vi "form status alarm string.vi"(0 "Vmon":dbl[][](array[numeric]), 1 "Vset":dbl[][](array[numeric]), 2 "Imon":dbl[][](array[numeric]), 3 "Iset":dbl[][](array[numeric]), 4 "Timestamps":dbl[][](array[numeric]), 5 "error in":errorcluster, 10 "Num Channels Read":i32, 12 "Start index":i32) -> (14 "Error Status String":string, 15 "All channels in error":string, 16 "Error Logged":bool[](array[boolean]), 17 "Error Array":string[][](array[string]), 18 "Status Strings":string[](array[string]), 19 "Error Out":errorcluster)   [LabVIEW 2018]
uses:
  CAEN globals.vi
  <userlib>/_OpenG.lib/array/array.llb/Search 1D Array (Boolean)__ogtk.vi
  <userlib>/_OpenG.lib/array/array.llb/Index 1D Array Elements (Boolean)__ogtk.vi
  <userlib>/_OpenG.lib/array/array.llb/Index 1D Array Elements (DBL)__ogtk.vi
  <userlib>/_OpenG.lib/array/array.llb/Index 1D Array Elements (String)__ogtk.vi
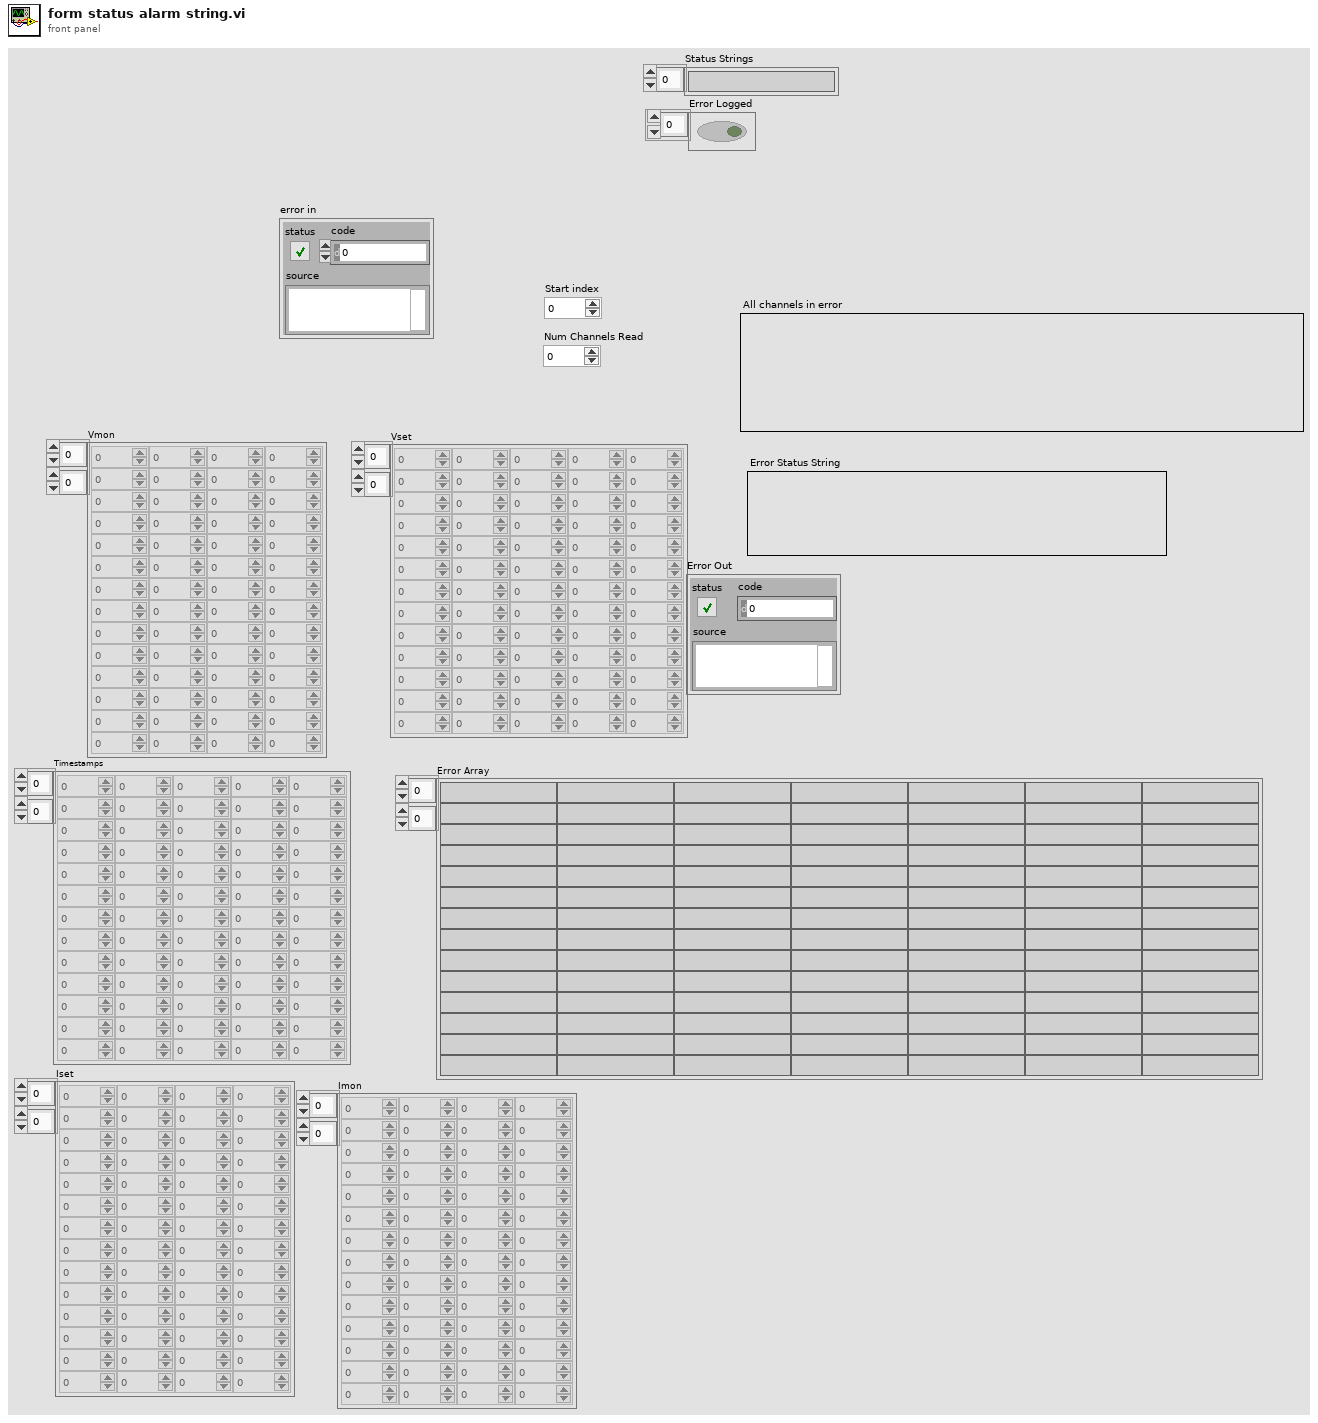
[diagram p1: front panel]
types:
  T1 = cluster{"Crate num":i32, "Slot nums":i32[], "Channel nums":i32[][], "N chans":i32[]}[]
  T2 = typedef "channel_cluster.ctl" = cluster{"Channel Name":string, "Crate":i32, "Card Type":string, "Card":i32, "Channel":i32, "Status Icon":picture, "Vmon (V)":dbl, "Vset (V)":dbl, "Imon (A)":dbl, "Iset (A)":dbl, "Timestamp":string, "ON/OFF":bool, "Status":string, "Vswmax (V)":dbl, "Flag":bool, "Vfile (V)":dbl, "Error Logged":bool[], "enable_file":bool}
  T3 = cluster{"Numeric":i32, "Indices of Elements":i32[], "Indices of Elements":i32[][], "Indices of Elements":i32[]}
  T4 = cluster{"Numeric":i32, "Indices of Elements":i32[], "Indices of Elements":i32[][], "Indices of Elements":i32[]}[]
  T5 = cluster{"Numeric":i32, "Indices of Elements":i32[], i32[][], i32[]}
  T6 = cluster{"Numeric":i32, "Indices of Elements":i32[], "Channel nums":i32[][], "N chans":i32[]}[]
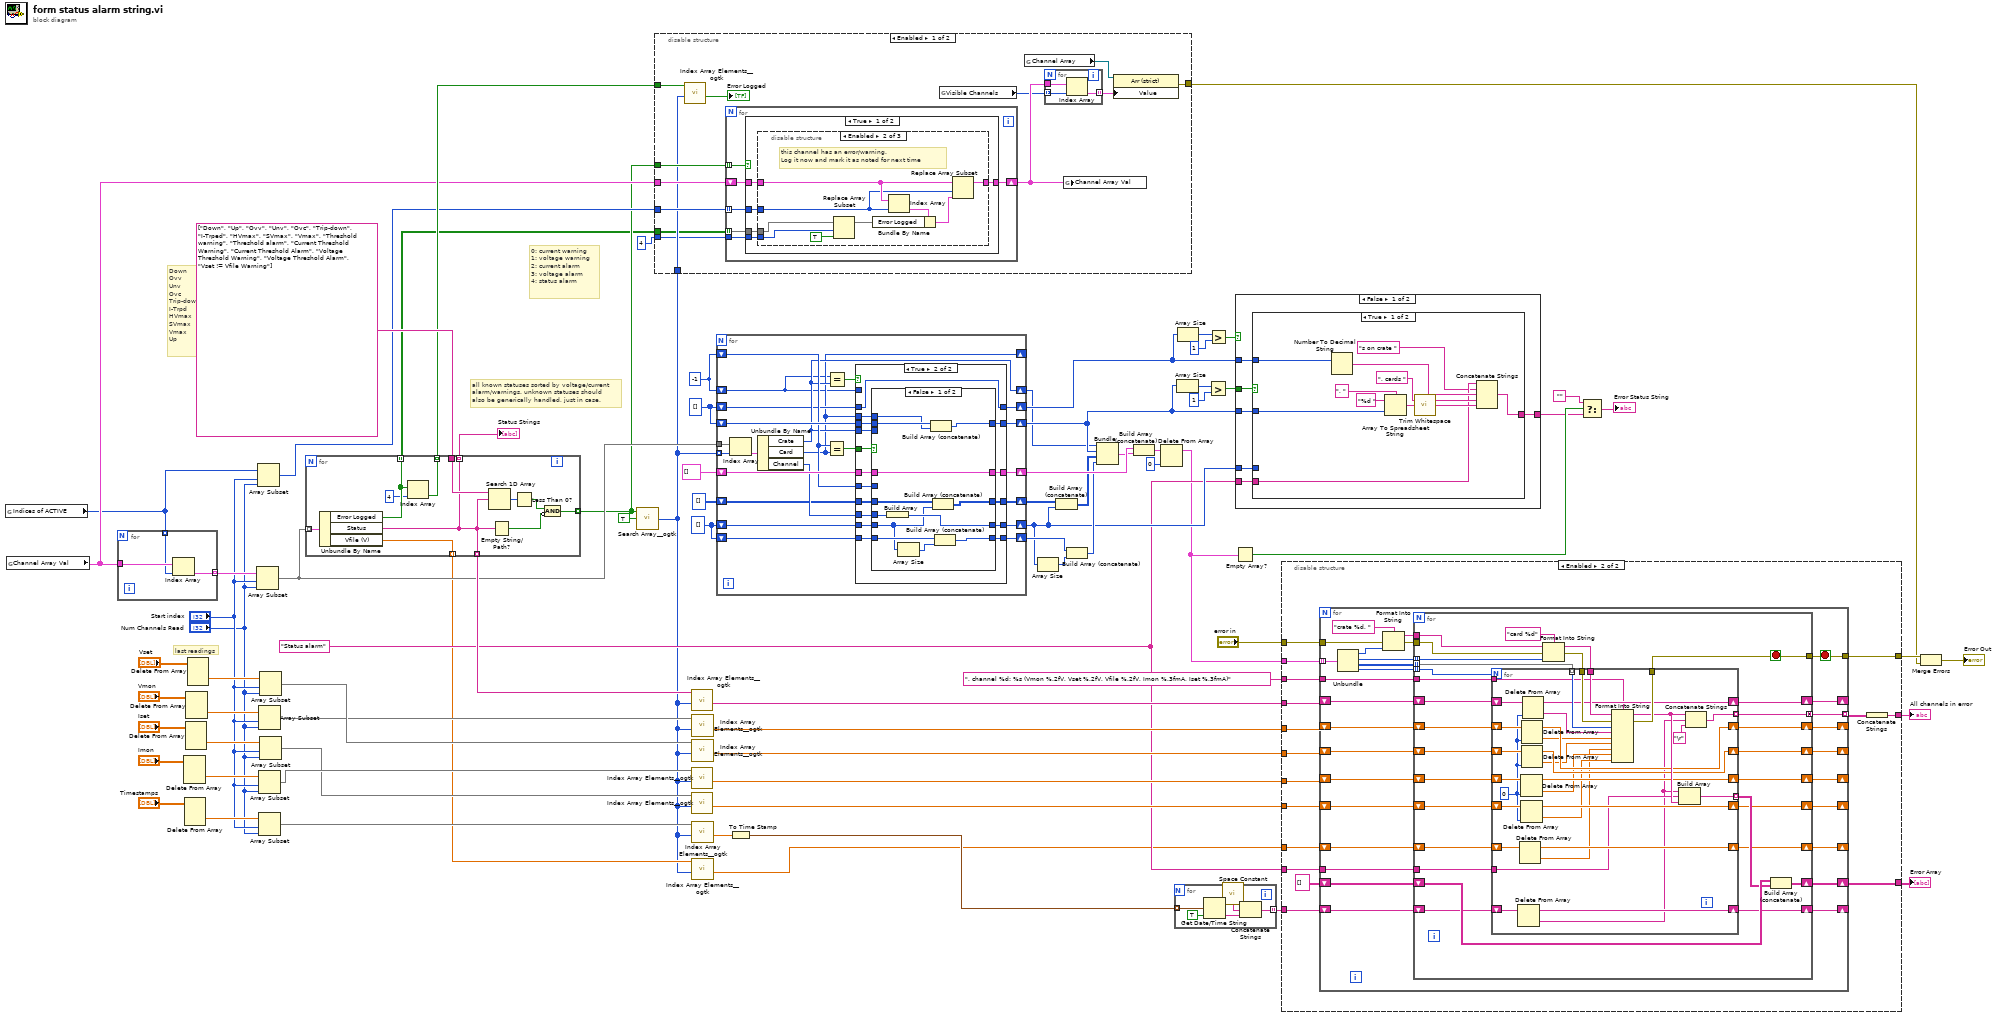
[diagram p0: block diagram]
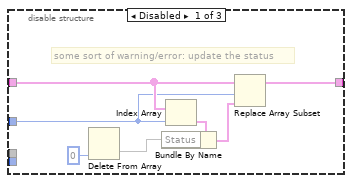
[diagram p2: hidden frame]
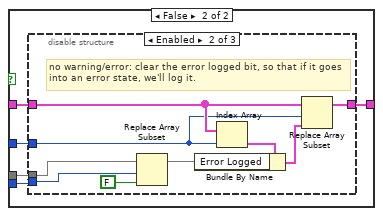
[diagram p4: hidden frame]
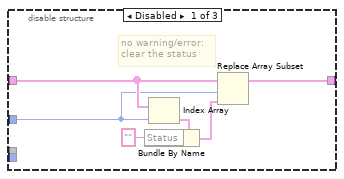
[diagram p5: hidden frame]
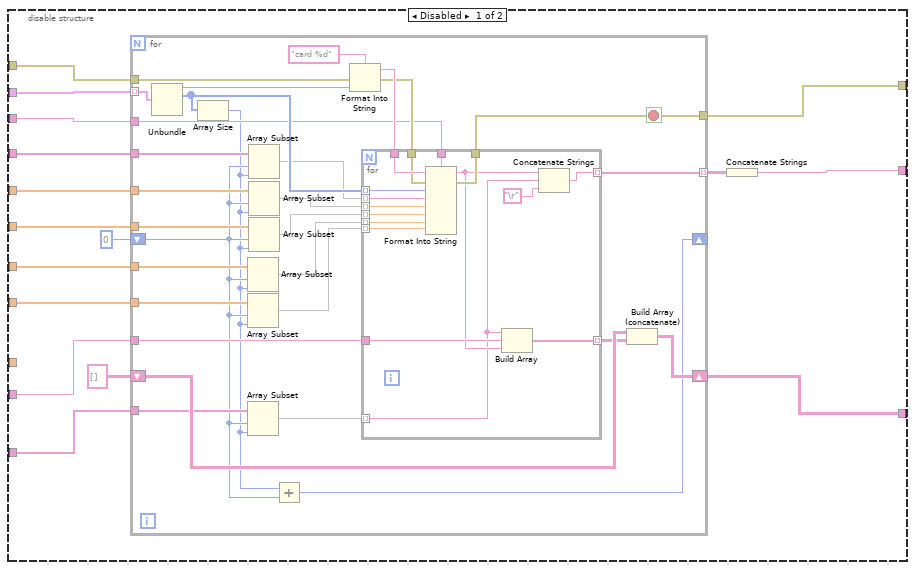
[diagram p8: hidden frame]
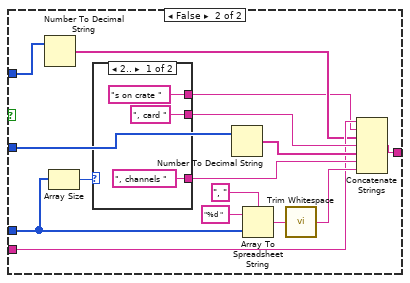
[diagram p9: hidden frame]
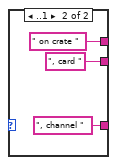
[diagram p10: hidden frame]
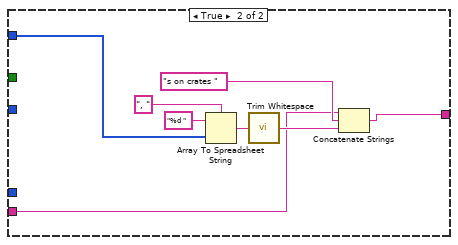
[diagram p11: hidden frame]
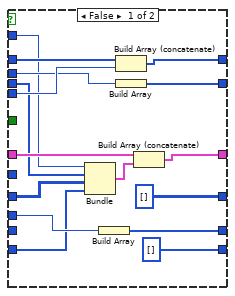
[diagram p12: hidden frame]
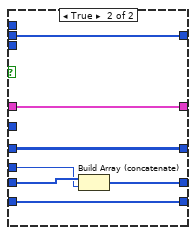
[diagram p13: hidden frame]
diagram:
  w24 = i32[] [] ("Indices of Elements")
  w37 = i32[] [] ("Indices of Elements")
  w26 = -1 ("Numeric")
  w21 = "Status alarm" ("Card type")
  # "0: current warning\n1: voltage warning\n2: current alarm\n3: voltage alarm\n4: status alarm"
  # "all known statuses sorted by voltage/current\nalarm/warnings. unknown statuses should\nalso be generically handled, just in case."
  # "Down\nOvv\nUnv\nOvc\nTrip-down\nI-Trpd\nHVmax\nSVmax\nVmax\nUp"
  # "last readings"
  n1 = global read "CAEN globals.vi" "Indices of ACTIVE"() -> (w10:i32[])
  n2 = global read "CAEN globals.vi" "Channel Array Val"() -> (w11:T2[])
  n3 = for {
    tunnel: w11 -> [w81]
    tunnel: [w80] -> w57 mode=indexing
    tunnel: w10 -> [w79] mode=indexing
    n4 = Index Array(array=w81, index=w79) -> (element=w80:T2)
  }
  n5 = Delete From Array(array="Imon") -> (deleted portion=w55:dbl[])  [unwired: 3 in, 1 out]
  n6 = Delete From Array(array="Timestamps") -> (deleted portion=w59:dbl[])  [unwired: 3 in, 1 out]
  n7 = Delete From Array(array="Iset") -> (deleted portion=w54:dbl[])  [unwired: 3 in, 1 out]
  n8 = Delete From Array(array="Vmon") -> (deleted portion=w61:dbl[])  [unwired: 3 in, 1 out]
  n9 = Delete From Array(array="Vset") -> (deleted portion=w63:dbl[])  [unwired: 3 in, 1 out]
  n10 = Array Subset(array=w57, index="Start index", length="Num Channels Read") -> (w27:T2[])
  n11 = Array Subset(array=w10, index="Start index", length="Num Channels Read") -> (w7:i32[])
  n12 = Array Subset(array=w61, index="Start index", length="Num Channels Read") -> (w60:dbl[])
  n13 = Array Subset(array=w55, index="Start index", length="Num Channels Read") -> (w50:dbl[])
  n14 = Array Subset(array=w59, index="Start index", length="Num Channels Read") -> (w58:dbl[])
  n15 = Array Subset(array=w63, index="Start index", length="Num Channels Read") -> (w62:dbl[])
  n16 = Array Subset(array=w54, index="Start index", length="Num Channels Read") -> (w49:dbl[])
  n17 = for {
    tunnel: w27 -> [w92] mode=indexing
    tunnel: [w88] -> w6 mode=indexing
    tunnel: [w85] -> w67 mode=indexing
    tunnel: string[] ["Down", "Up", "Ovv", "Unv", "Ovc", "Trip-down", "I-Trped", "HVmax", "SVmax", "Vmax", "Threshold warning", "Threshold alarm", "Current Threshold Warning", "Current Threshold Alarm", "Voltage Threshold Warning", "Voltage Threshold Alarm", "Vset != Vfile Warning"] -> [w87]
    tunnel: [w86] -> w16 mode=indexing
    tunnel: [w85] -> w14 mode=indexing
    tunnel: [w84] -> w13 mode=indexing
    tunnel: [w83] -> w5 mode=indexing
    n18 = Unbundle By Name(w92) -> ("Error Logged"=w83:bool[], "Status"=w85:string, "Vfile (V)"=w86:dbl)
    n19 = Index Array(array=w83, index=4 ("Numeric")) -> (element=w84:bool)
    n20 = Search 1D Array(1D array=w87, element=w85) -> (index of element=w91:i32)  [unwired: 1 in]
    n21 = Empty String/Path?(string/path=w85) -> (empty?=w89:bool)
    n22 = Less Than 0?(x=w91) -> (x < 0?=w90:bool)
    n23 = Compound Arithmetic op=AND(w90, invert w89) -> (w88:bool)
  }
  "Status Strings" <- w14
  n24 = call-poly <userlib>:"Search Array__ogtk.vi"("Array"=w6, "Element Data"=TRUE) -> ("Indices of Elements"=w12:i32[])  [unwired: 7 in]
  n25 = disable-structure shown="Enabled" {
    disable-tunnel: [w105 _] -> w2
    disable-tunnel: w11 -> [w100 _]
    disable-tunnel: w12 -> [w97 _]
    disable-tunnel: w7 -> [w99 _]
    disable-tunnel: w6 -> [w98 _]
    disable-tunnel: w13 -> [w96 _]
    disable-tunnel: w5 -> [w95 _]
    disable-tunnel: 4 ("Numeric") -> [w94 _]
    frame Enabled {
      n26 = call-poly <userlib>:"Index Array Elements__ogtk.vi"("indices"=w97, "array"=w96) -> ("elements"=→"Error Logged":bool[])  [unwired: 9 in]
      n27 = for {
        shift-right: [w112] -> w104
        shift-left: w100 -> [w114]
        tunnel: w99 -> [w113] mode=indexing
        tunnel: w98 -> [w111] mode=indexing
        tunnel: w95 -> [w110] mode=indexing
        tunnel: w94 -> [w109]
        n28 = case shown="True" w111 {
          tunnel: w114 -> [w119 w142]
          tunnel: w113 -> [w118 w141]
          tunnel: [w117 w140] -> w112
          tunnel: w110 -> [w116 w139]
          tunnel: w109 -> [w115 w138]
          frame True {
            n29 = disable-structure shown="Enabled" {
              disable-tunnel: w119 -> [w128 w137 _]
              disable-tunnel: w118 -> [w127 w136 _]
              disable-tunnel: [w126 w135 _] -> w117
              disable-tunnel: w116 -> [_ w132 _]
              disable-tunnel: w115 -> [_ w131 _]
              frame Disabled {
                # "some sort of warning/error: update the status"
                n30 = Delete From Array(index=0) -> (deleted portion=w122, array=w125:string[], array with subset deleted=w124)  [unwired: 1 in]
                n31 = Index Array(array=w128, index=w127) -> (element=w121:T2)
                n32 = Bundle By Name(cluster=w121, "Status"=w122) -> (w120:T2)
                n33 = Replace Array Subset(array=w128, new element=w120, index=w127) -> (w126:T2[])
              }
              frame Enabled {
                # "this channel has an error/warning. \nLog it now and mark it as noted for next time"
                n34 = Replace Array Subset(array=w132, new element=TRUE ("Element Data"), index=w131) -> (w130:bool[])
                n35 = Index Array(array=w137, index=w136) -> (element=w134:T2)
                n36 = Bundle By Name(cluster=w134, "Error Logged"=w130) -> (w133:T2)
                n37 = Replace Array Subset(array=w137, new element=w133, index=w136) -> (w135:T2[])
              }
              frame Disabled {
              }
            }
          }
          frame False {
            n38 = disable-structure shown="Enabled" {
              disable-tunnel: w142 -> [w148 w157 _]
              disable-tunnel: w141 -> [w147 w156 _]
              disable-tunnel: [w146 w155 _] -> w140
              disable-tunnel: w139 -> [_ w151 _]
              disable-tunnel: w138 -> [_ w150 _]
              frame Disabled {
                # "no warning/error:\nclear the status"
                n39 = Index Array(array=w148, index=w147) -> (element=w145:T2)
                n40 = Bundle By Name(cluster=w145, "Status"="") -> (w144:T2)
                n41 = Replace Array Subset(array=w148, new element=w144, index=w147) -> (w146:T2[])
              }
              frame Enabled {
                # "no warning/error: clear the error logged bit, so that if it goes into an error state, we'll log it."
                n42 = Replace Array Subset(array=w151, new element=FALSE ("Element Data"), index=w150) -> (w152:bool[])
                n43 = Index Array(array=w157, index=w156) -> (element=w154:T2)
                n44 = Bundle By Name(cluster=w154, "Error Logged"=w152) -> (w153:T2)
                n45 = Replace Array Subset(array=w157, new element=w153, index=w156) -> (w155:T2[])
              }
              frame Disabled {
              }
            }
          }
        }
      }
      n46 = global read "CAEN globals.vi" "Visible Channels"() -> (w103:i32[])
      n47 = global read "CAEN globals.vi" "Channel Array"() -> (w102:refnum<vi>)
      n48 = for {
        tunnel: w104 -> [w108]
        tunnel: w103 -> [w107] mode=indexing
        tunnel: [w106] -> w101 mode=indexing
        n49 = Index Array(array=w108, index=w107) -> (element=w106:T2)
      }
      n50 = global write "CAEN globals.vi" "Channel Array Val"(w104) -> ()
      n51 = property class="Arr (strict)"(reference=w102, "Value"=w101) -> (error out=w105:errorcluster)  [unwired: 1 in, 1 out]
    }
    frame Disabled {
    }
  }
  n52 = call-poly <userlib>:"Index Array Elements__ogtk.vi"("indices"=w12, "array"=w67) -> ("elements"=w56:string[])  [unwired: 9 in]
  n53 = call-poly <userlib>:"Index Array Elements__ogtk.vi"("indices"=w12, "array"=w50) -> ("elements"=w47:dbl[])  [unwired: 9 in]
  n54 = call-poly <userlib>:"Index Array Elements__ogtk.vi"("indices"=w12, "array"=w49) -> ("elements"=w46:dbl[])  [unwired: 9 in]
  n55 = call-poly <userlib>:"Index Array Elements__ogtk.vi"("indices"=w12, "array"=w60) -> ("elements"=w70:dbl[])  [unwired: 9 in]
  n56 = call-poly <userlib>:"Index Array Elements__ogtk.vi"("indices"=w12, "array"=w62) -> ("elements"=w51:dbl[])  [unwired: 9 in]
  n57 = call-poly <userlib>:"Index Array Elements__ogtk.vi"("indices"=w12, "array"=w58) -> ("elements"=w68:dbl[])  [unwired: 9 in]
  n58 = call-poly <userlib>:"Index Array Elements__ogtk.vi"("indices"=w12, "array"=w16) -> ("elements"=w15:dbl[])  [unwired: 9 in]
  n59 = for {
    tunnel: w12 -> [w174] mode=indexing
    shift-right: [w164] -> _
    shift-left: w26 -> [w170]
    shift-right: [w179] -> w34
    shift-left: i32[][] [] ("Indices of Elements") -> [w160]
    shift-right: [w178] -> w40
    shift-left: T1 [] -> [w177]
    shift-right: [w175] -> w31
    shift-left: w37 -> [w176]
    tunnel: w27 -> [w173]
    shift-right: [w167] -> w22
    shift-left: w26 -> [w163]
    shift-right: [w165] -> w32
    shift-left: w37 -> [w166]
    shift-right: [w161] -> w23
    shift-left: w24 -> [w162]
    shift-right: [w158] -> w29
    shift-left: w24 -> [w159]
    n60 = Index Array(array=w173, index=w174) -> (element=w172:T2)
    n61 = Unbundle By Name(w172) -> ("Crate"=w167:i32, "Card"=w164:i32, "Channel"=w171:i32)
    n62 = Equal?(x=w170, y=w164) -> (x = y?=w168:bool)
    n63 = Equal?(x=w163, y=w167) -> (x = y?=w169:bool)
    n64 = case shown="True" w169 {
      tunnel: w160 -> [w184 w211]
      tunnel: [i32[][] [] ("Indices of Elements") w210] -> w179
      tunnel: [w191 w209] -> w178
      tunnel: w177 -> [w192 w208]
      tunnel: w176 -> [w185 w207]
      tunnel: [w187 w206] -> w175
      tunnel: w171 -> [w189 w205]
      tunnel: w170 -> [_ w204]
      tunnel: w168 -> [_ w203]
      tunnel: w167 -> [w190 w202]
      tunnel: w166 -> [w195 w201]
      tunnel: [w194 w201] -> w165
      tunnel: w164 -> [w188 w198]
      tunnel: w163 -> [w186 _]
      tunnel: w162 -> [_ w199]
      tunnel: [w183 w200] -> w161
      tunnel: w159 -> [w181 w197]
      tunnel: [i32[] [] ("Indices of Elements") w196] -> w158
      frame False {
        n65 = Bundle("Numeric"=w186, "Indices of Elements"=w185, "Indices of Elements"=w184, "Indices of Elements"=w181) -> (w193:T3)  [unwired: 1 in]
        n66 = Build Array(w189) -> (w183:i32[])
        n67 = Build Array (concatenate)(w195, w190) -> (w194:i32[])
        n68 = Build Array(w188) -> (w187:i32[])
        n69 = Build Array (concatenate)(w192, w193) -> (w191:T4)
      }
      frame True {
        n70 = case shown="False" w203 {
          tunnel: w211 -> [w217 w228]
          tunnel: w205 -> [w220 w226]
          tunnel: [w223 w228] -> w210
          tunnel: [w219 w230] -> w209
          tunnel: w208 -> [w219 w230]
          tunnel: w204 -> [_ _]
          tunnel: w207 -> [w221 w229]
          tunnel: [w222 w229] -> w206
          tunnel: w202 -> [_ _]
          tunnel: [w218 w225] -> w200
          tunnel: w199 -> [w212 w227]
          tunnel: w198 -> [w216 _]
          tunnel: w197 -> [w215 w224]
          tunnel: [w214 w224] -> w196
          frame False {
            n71 = Build Array(w220) -> (w218:i32[])
            n72 = Array Size(array=w212) -> (size(s)=w213:i32)
            n73 = Build Array (concatenate)(w221, w216) -> (w222:i32[])
            n74 = Build Array (concatenate)(w217, w212) -> (w223:i32[][])
            n75 = Build Array (concatenate)(w215, w213) -> (w214:i32[])
          }
          frame True {
            n76 = Build Array (concatenate)(w227, w226) -> (w225:i32[])
          }
        }
      }
    }
  }
  n77 = To Time Stamp(1:w68) -> (0:w65:timestamp[])
  n78 = Array Size(array=w23) -> (size(s)=w30:i32)
  n79 = Build Array (concatenate)(w34, w23) -> (w33:i32[][])
  n80 = Build Array (concatenate)(w29, w30) -> (w28:i32[])
  n81 = Bundle("Numeric"=w22, "Indices of Elements"=w31, w33, w28) -> (w39:T5)  [unwired: 1 in]
  n82 = Build Array (concatenate)(w40, w39) -> (w38:T6)
  n83 = Delete From Array(array=w38, index=0) -> (array with subset deleted=w20:T6)  [unwired: 1 in, 1 out]
  n84 = for {
    tunnel: w65 -> [w232] mode=indexing
    tunnel: [w231] -> w64 mode=indexing
    n85 = Get Date/Time String(seconds (now)=w232, want seconds? (F)=TRUE) -> (date string=w235:string, time string=w233:string)  [unwired: 1 in]
    n86 = call <vilib>:"Space Constant.vi"() -> ("String"=w236:string)
    n87 = Concatenate Strings(w235, w236, w233) -> (w231:string)
  }
  n88 = Array Size(array=w31) -> (size(s)=w44:i32)
  n89 = Array Size(array=w32) -> (size(s)=w35:i32)
  n90 = Greater?(x=w44, y=1) -> (0:w19:bool)
  n91 = Greater?(x=w35, y=1) -> (0:w18:bool)
  n92 = Empty Array?(array=w20) -> (empty?=w78:bool)
  n93 = case shown="False" w18 {
    tunnel: w19 -> [w242 _]
    tunnel: w23 -> [w241 _]
    tunnel: w31 -> [w240 _]
    tunnel: [w239 w277] -> w17
    tunnel: w21 -> [w238 w276]
    tunnel: w32 -> [w237 w275]
    frame False {
      n94 = case shown="True" w242 {
        tunnel: w240 -> [w248 w267]
        tunnel: [w252 w268] -> w239
        tunnel: w241 -> [_ w266]
        tunnel: w238 -> [w244 w257]
        tunnel: w237 -> [w245 w255]
        frame True {
          n95 = Number To Decimal String(number=w245) -> (decimal integer string=w246:string[])  [unwired: 1 in]
          n96 = Array To Spreadsheet String(delimiter (Tab)=", ", array=w248, 3:"%d " ("delimiter (Tab)")) -> (spreadsheet string=w250:string)
          n97 = call <vilib>:"Trim Whitespace.vi"("string"=w250) -> ("trimmed string"=w249:string)  [unwired: 1 in]
          n98 = Concatenate Strings(w244, "s on crate " ("Card type"), w246, ", cards " ("Card type"), w249) -> (w252:string)
        }
        frame False {
          n99 = Number To Decimal String(number=w255) -> (decimal integer string=w256:string[])  [unwired: 1 in]
          n100 = Array Size(array=w266) -> (size(s)=w260:i32)
          n101 = case shown="2.." w260 {
            tunnel: [", channels " ("Card type") ", channel " ("Card type")] -> w259
            tunnel: [", card " ("Card type") ", card " ("Card type")] -> w258
            tunnel: ["s on crate " ("Card type") " on crate " ("Card type")] -> w254
            frame 2.. {
            }
            frame ..1 {
            }
          }
          n102 = Number To Decimal String(number=w267) -> (decimal integer string=w262:string[])  [unwired: 1 in]
          n103 = Array To Spreadsheet String(delimiter (Tab)=", ", array=w266, 3:"%d " ("delimiter (Tab)")) -> (spreadsheet string=w264:string)
          n104 = call <vilib>:"Trim Whitespace.vi"("string"=w264) -> ("trimmed string"=w263:string)  [unwired: 1 in]
          n105 = Concatenate Strings(w257, w254, w256, w258, w262, w259, w263) -> (w268:string)
        }
      }
    }
    frame True {
      n106 = Array To Spreadsheet String(delimiter (Tab)=", ", array=w275, 3:"%d " ("delimiter (Tab)")) -> (spreadsheet string=w282:string)
      n107 = call <vilib>:"Trim Whitespace.vi"("string"=w282) -> ("trimmed string"=w281:string)  [unwired: 1 in]
      n108 = Concatenate Strings(w276, "s on crates " ("Card type"), w281) -> (w277:string)
    }
  }
  n109 = disable-structure shown="Enabled" {
    disable-tunnel: [w297 w346] -> w73
    disable-tunnel: [w295 w347] -> w72
    disable-tunnel: w70 -> [w293 w355]
    disable-tunnel: "error in" -> [w292 w358]
    disable-tunnel: w64 -> [w291 w348]
    disable-tunnel: w56 -> [w290 w352]
    disable-tunnel: [w289 w344] -> w3
    disable-tunnel: w51 -> [w288 w354]
    disable-tunnel: ", channel %d: %s (Vmon %.2fV, Vset %.2fV, Vfile %.2fV, Imon %.3fmA, Iset %.3fmA)" ("delimiter (Tab)") -> [w287 w356]
    disable-tunnel: w47 -> [w286 w351]
    disable-tunnel: w46 -> [w285 w350]
    disable-tunnel: w21 -> [w284 w353]
    disable-tunnel: w20 -> [w283 w357]
    disable-tunnel: w15 -> [_ w349]
    frame Disabled {
      n110 = for {
        tunnel: w293 -> [w318]
        tunnel: w288 -> [w316]
        tunnel: w283 -> [w322] mode=indexing
        tunnel: w287 -> [w306]
        tunnel: [w326] -> w298 mode=indexing
        shift-right: [w325] -> w295
        shift-left: string[][] [] -> [w324]
        tunnel: w284 -> [w305]
        shift-right: [w314] -> _
        shift-left: 0 -> [w302]
        tunnel: w292 -> [w313]
        tunnel: [w311] -> w289
        tunnel: w291 -> [w308]
        tunnel: w290 -> [w310]
        tunnel: w286 -> [w304]
        tunnel: w285 -> [w303]
        stop <- w311 stop-if-true
        n111 = Unbundle(w322) -> ("Numeric"=w321:i32, "Indices of Elements"=w319:i32[])  [unwired: 2 out]
        n112 = Array Size(array=w319) -> (size(s)=w301:i32)
        n113 = Array Subset(array=w304, index=w302, length=w301) -> (w300:dbl[])
        n114 = Array Subset(array=w303, index=w302, length=w301) -> (w299:dbl[])
        n115 = Array Subset(array=w308, index=w302, length=w301) -> (w307:string[])
        n116 = Array Subset(array=w310, index=w302, length=w301) -> (w309:string[])
        n117 = Array Subset(array=w318, index=w302, length=w301) -> (w317:dbl[])
        n118 = Array Subset(array=w316, index=w302, length=w301) -> (w315:dbl[])
        n119 = Add(x=w301, y=w302) -> (x+y=w314:i32)
        n120 = Format Into String(format string="card %d" ("Card type"), error in=w313, w321) -> (resulting string=w327:string, error out=w312:errorcluster)  [unwired: 1 in]
        n121 = for {
          tunnel: w319 -> [w337] mode=indexing
          tunnel: w317 -> [w340] mode=indexing
          tunnel: w315 -> [w339] mode=indexing
          tunnel: w306 -> [w343]
          tunnel: w327 -> [w342]
          tunnel: [w332] -> w326 mode=indexing
          tunnel: [w341] -> w311
          tunnel: [w338] -> w323 mode=indexing
          tunnel: w305 -> [w335]
          tunnel: w312 -> [w336]
          tunnel: w307 -> [w331] mode=indexing
          tunnel: w309 -> [w328] mode=indexing
          tunnel: w300 -> [w330] mode=indexing
          tunnel: w299 -> [w329] mode=indexing
          n122 = Format Into String(format string=w343, initial string=w342, error in=w336, w337, w328, w340, w339, w330, w329) -> (resulting string=w334:string, error out=w341:errorcluster)
          n123 = Build Array(w331, w335, w334) -> (w338:string[])
          n124 = Concatenate Strings(w334, w331, "\r") -> (w332:string)
        }
        n125 = Build Array (concatenate)(w324, w323) -> (w325:string[][])
      }
      n126 = Concatenate Strings(w298) -> (w297:string)
    }
    frame Enabled {
      n127 = for {
        tunnel: [w388] -> w345 mode=indexing
        tunnel: w357 -> [w382] mode=indexing
        tunnel: w356 -> [w385]
        tunnel: w358 -> [w381]
        tunnel: [w383] -> w344
        shift-right: [w386] -> w347
        shift-left: string[][] [] -> [w387]
        shift-right: [w369] -> _
        shift-left: w352 -> [w376]
        shift-right: [w366] -> _
        shift-left: w355 -> [w375]
        shift-right: [w367] -> _
        shift-left: w354 -> [w374]
        shift-right: [w370] -> _
        shift-left: w351 -> [w373]
        shift-right: [w368] -> _
        shift-left: w350 -> [w384]
        shift-right: [w363] -> _
        shift-left: w349 -> [w364]
        tunnel: w353 -> [w362]
        shift-right: [w360] -> _
        shift-left: w348 -> [w361]
        stop <- w383 stop-if-true
        n128 = Unbundle(w382) -> ("Numeric"=w378:i32, "Indices of Elements"=w372:i32[], "Channel nums"=w371:i32[][], "N chans"=w365:i32[])
        n129 = Format Into String(format string="crate %d, " ("Card type"), error in=w381, w378) -> (resulting string=w377:string, error out=w380:errorcluster)  [unwired: 1 in]
        n130 = for {
          tunnel: w385 -> [w398]
          tunnel: [w416] -> w388 mode=concatenating
          shift-right: [w415] -> w386
          shift-left: w387 -> [w414]
          tunnel: w380 -> [w411]
          tunnel: [w409] -> w383
          tunnel: w372 -> [w408] mode=indexing
          tunnel: w371 -> [w402] mode=indexing
          tunnel: w377 -> [w407]
          shift-right: [w405] -> w370
          shift-left: w373 -> [w406]
          shift-right: [w390] -> w367
          shift-left: w374 -> [w393]
          shift-right: [w389] -> w366
          shift-left: w375 -> [w394]
          shift-right: [w395] -> w369
          shift-left: w376 -> [w396]
          shift-right: [w403] -> w368
          shift-left: w384 -> [w404]
          tunnel: w365 -> [w401] mode=indexing
          shift-right: [w399] -> w363
          shift-left: w364 -> [w400]
          tunnel: w362 -> [w397]
          shift-right: [w391] -> w360
          shift-left: w361 -> [w392]
          stop <- w409 stop-if-true
          n131 = Format Into String(format string="card %d" ("Card type"), initial string=w407, error in=w411, w408) -> (resulting string=w417:string, error out=w410:errorcluster)
          n132 = for {
            N: w401 -> [_]
            tunnel: w402 -> [w446] mode=indexing
            tunnel: w417 -> [w449]
            tunnel: [w442] -> w416 mode=indexing
            tunnel: [w448] -> w409
            tunnel: [w447] -> w413 mode=indexing
            tunnel: w410 -> [w445]
            shift-right: [w440] -> w405
            shift-left: w406 -> [w441]
            shift-right: [w434] -> w395
            shift-left: w396 -> [w438]
            shift-right: [w435] -> w389
            shift-left: w394 -> [w437]
            shift-right: [w436] -> w390
            shift-left: w393 -> [w439]
            shift-right: [w431] -> w403
            shift-left: w404 -> [w433]
            shift-right: [w429] -> w399
            shift-left: w400 -> [w430]
            tunnel: w398 -> [w428]
            tunnel: w397 -> [w427]
            shift-right: [w419] -> w391
            shift-left: w392 -> [w420]
            w432 = 0 ("index")
            n133 = Delete From Array(array=w420) -> (deleted portion=w418:string, array with subset deleted=w419:string[])  [unwired: 2 in]
            n134 = Delete From Array(array=w430) -> (deleted portion=w421:dbl, array with subset deleted=w429:dbl[])  [unwired: 2 in]
            n135 = Delete From Array(array=w441, index=w432) -> (deleted portion=w422:dbl, array with subset deleted=w440:dbl[])  [unwired: 1 in]
            n136 = Delete From Array(array=w433, index=w432) -> (deleted portion=w423:dbl, array with subset deleted=w431:dbl[])  [unwired: 1 in]
            n137 = Delete From Array(array=w437, index=w432) -> (deleted portion=w425:dbl, array with subset deleted=w435:dbl[])  [unwired: 1 in]
            n138 = Delete From Array(array=w439, index=w432) -> (deleted portion=w424:dbl, array with subset deleted=w436:dbl[])  [unwired: 1 in]
            n139 = Delete From Array(array=w438, index=w432) -> (deleted portion=w426:string, array with subset deleted=w434:string[])  [unwired: 1 in]
            n140 = Format Into String(format string=w428, initial string=w449, error in=w445, w446, w426, w425, w424, w421, w422, w423) -> (resulting string=w444:string, error out=w448:errorcluster)
            n141 = Build Array(w418, w427, w444) -> (w447:string[])
            n142 = Concatenate Strings(w444, w418, "\r") -> (w442:string)
          }
          n143 = Build Array (concatenate)(w414, w413) -> (w415:string[][])
        }
      }
      n144 = Concatenate Strings(w345) -> (w346:string)
    }
  }
  "All channels in error" <- w73
  "Error Array" <- w72
  n145 = Select(t="", s=w78, f=w17) -> (s? t:f=→"Error Status String":string)
  n146 = Merge Errors(w3, w2) -> (→"Error Out":errorcluster)
